vi "Child Msgs.vi"(6 "Unified Actor Alias":string, 7 "Actor in":refnum<class "Actor.lvclass">) -> (0 "Error out":errorcluster, 2 "Msgs":T1)   [LabVIEW 2020, in "jettl.lvlib" / "Read Unified Actor.lvlib"]
uses:
  Read Unified Actor.lvlib
  Actor Specific/Actor Specific.lvlib
  Actor Specific/Find Child Attributes.vi
  Actor/Actor.lvclass
  Msg/Msg.lvclass
  Msg Set.ctl
  jettl.lvlib
  Msgs.ctl
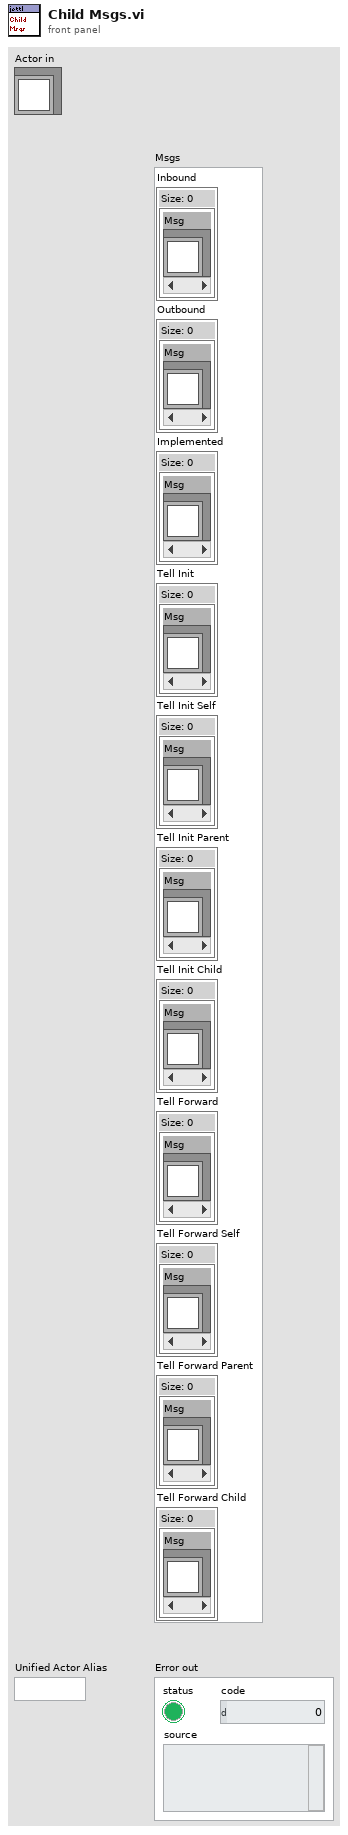
[diagram p1: front panel]
types:
  T1 = typedef "jettl.lvlib/Msgs.ctl" = cluster{"Inbound":T2, "Outbound":T2, "Implemented":T2, "Tell Init":T2, "Tell Init Self":T2, "Tell Init Parent":T2, "Tell Init Child":T2, "Tell Forward":T2, "Tell Forward Self":T2, "Tell Forward Parent":T2, "Tell Forward Child":T2}
  T2 = typedef "jettl.lvlib/Msg Set.ctl" = set{refnum<class "Msg.lvclass">}
  T3 = typedef "jettl.lvlib/Unified Actor.ctl" = cluster{"Msgs":T1, "Leaf":bool, "Edge Actors":refnum<class "Actor.lvclass">[], "Core Actors":refnum<class "Actor.lvclass">[], "Root":bool, "Alias":string, "DVR UID":i32, "Transport":refnum<user-event>, "Address":refnum<event-registration>, "This VI":refnum<vi>}
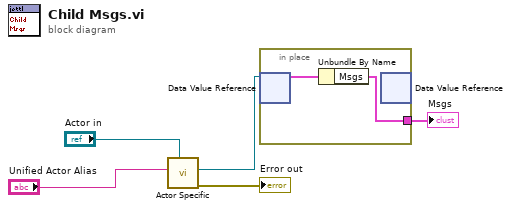
[diagram p0: block diagram]
diagram:
  n1 = call-poly "Actor Specific.vi"("Actor in"="Actor in", "Unified Actor Alias"="Unified Actor Alias") -> ("Error out"=→"Error out":errorcluster, "Child Unified Actor DVR"=w2:refnum<data-value>)  [unwired: 8 in]
  n2 = in-place {
    in-place-border: [w6] -> w5
    n3 = in-place-dvr #1(w2) -> (w7:T3)  [unwired: 1 out]
    n4 = Unbundle By Name(w7) -> ("Msgs"=w6:T1)
    n5 = in-place-dvr #1() -> ()  [unwired: 1 in, 2 out]
  }
  "Msgs" <- w5
